vi "01 DoubleCheck.vi"(8 "error in (no error)":errorcluster caption="错误输入（无错误）", 10 "串口配置":T1={"VISA串口名称"="", "波特率"=9600, "停止位"=10, "流控制"=0, "数据位"=8, "奇偶校验"=enum."None", "超时"=2000, "启用终止符？"=FALSE, "终止符"=10} {"终止符" format="%.0x"; "数据位" min=5 max=8 step=1; "流控制" items=["无", "XON/XOFF", "RTS/CTS", "XON/XOFF & RTS/CTS", "DTR/DSR", "XON/XOFF & DTR/DSR"]; "停止位" items=["1.0"=10, "1.5"=15, "2.0"=20]; "波特率" items=["9600"=9600, "115200"=15]}, 11 "SerialClass 输入":refnum<class "SerialClass.lvclass">) -> (0 "error out":errorcluster caption="错误输出", 1 "串口配置输出":T1={"VISA串口名称"="", "波特率"=9600, "停止位"=10, "流控制"=0, "数据位"=8, "奇偶校验"=enum."None", "超时"=2000, "启用终止符？"=FALSE, "终止符"=10} {"终止符" format="%.0x"; "数据位" min=5 max=8 step=1; "流控制" items=["无", "XON/XOFF", "RTS/CTS", "XON/XOFF & RTS/CTS", "DTR/DSR", "XON/XOFF & DTR/DSR"]; "停止位" items=["1.0"=10, "1.5"=15, "2.0"=20]; "波特率" items=["9600"=9600, "115200"=15]}, 2 "重复？":bool, 3 "SerialClass 输出":refnum<class "SerialClass.lvclass">)   [LabVIEW 2019, in "SerialClass.lvclass"]
uses:
  SerialClass.lvclass
  00 Ctl/SerialData.ctl
  SerialClass.lvclass/SerialClass.ctl
panel:
  # "重复检查"
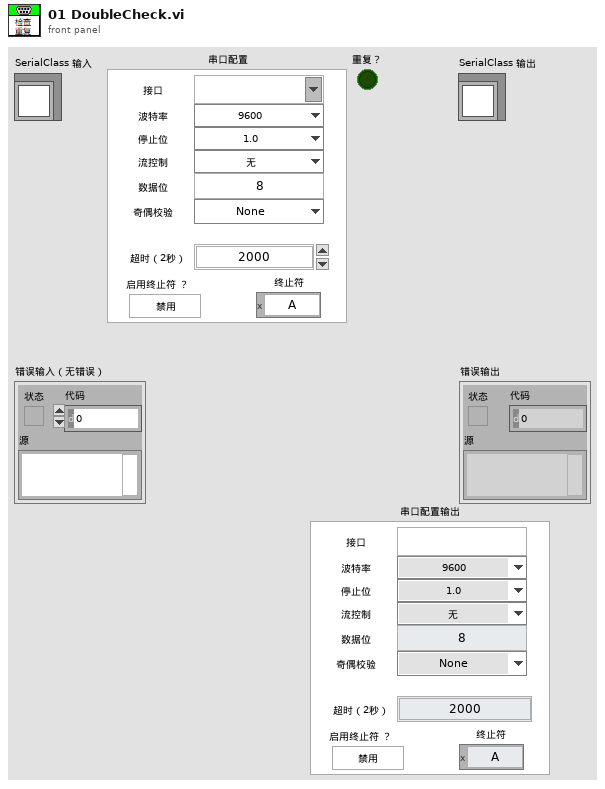
[diagram p1: front panel]
types:
  T1 = typedef "SerialData.ctl" = cluster{"VISA串口名称":refnum<visa-resource-name>, "波特率":u32, "停止位":u16, "流控制":u16, "数据位":u16, "奇偶校验":enum16{"None", "Odd", "Even", "Mark", "Space"}, "超时":u32, "启用终止符？":bool, "终止符":u8}
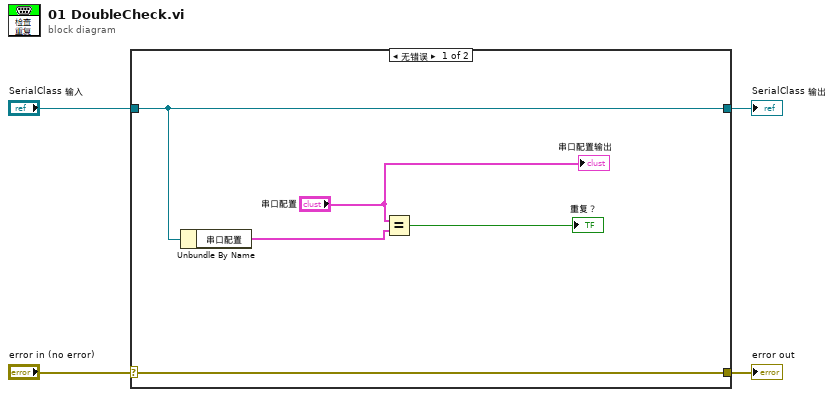
[diagram p0: block diagram]
diagram:
  n1 = case shown="无错误" "error in (no error)" {
    selector: "error in (no error)" -> [w9 w11]
    tunnel: [w9 w11] -> w3
    tunnel: [w6 w10] -> w1
    tunnel: "SerialClass 输入" -> [w6 w10]
    frame No Error {
      n2 = Unbundle By Name(w6) -> ("串口配置"=w8:T1)
      n3 = Equal?(x="串口配置", y=w8) -> (x = y?=→"重复？":bool)
      "串口配置输出" <- "串口配置"
    }
    frame Error {
    }
  }
  "error out" <- w3
  "SerialClass 输出" <- w1
